vi "Asynchronous Call and Forget.vi"   [LabVIEW 2019]
doc: "This VI demonstrates an asynchronous call and forget. When this VI is run, it asynchronously calls a target VI and will not wait for the results. This VI will run to completion while the target VI continues to run.\n\nThis example uses the Start Asynchronous Call method and the Open VI Reference option 0x80.\n\nWhen running this example, notice this VI finishes execution while the target VI continues to run."
panel:
  # "Overview: Demonstrates the use of the call and forget option (0x80) with Asynchronous VI Calls.\nInstructions:\nRun the VI. Observe the behavior of the VI being called asynchronously, and notice that this VI stops running, even when the asynchronous VI is still running. See the block diagram for more information."
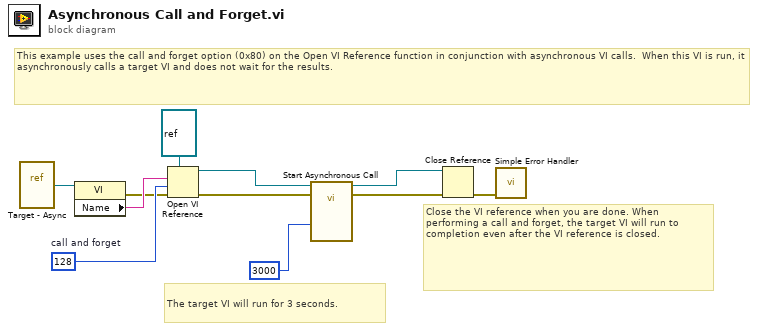
[diagram p0: block diagram]
diagram:
  w11 = 128  # call and forget
  # "This example uses the call and forget option (0x80) on the Open VI Reference function in conjunction with asynchronous VI calls.  When this VI is run, it asynchronously calls a target VI and does not wait for the results."
  # "Close the VI reference when you are done. When performing a call and forget, the target VI will run to completion even after the VI reference is closed."
  # "The target VI will run for 3 seconds."
  n1 = vi-ref "Target - Async.vi"() -> (w4:refnum<vi>)
  n2 = property class="VI"(reference=w4) -> (error out=w1:errorcluster, "Name"=w3:string)  [unwired: 1 in, 1 out]
  n3 = Open VI Reference(type specifier VI Refnum (for type only)=refnum<vi> refnum, vi path=w3, options=w11, error in (no error)=w1) -> (vi reference=w9:refnum<vi>, error out=w8:errorcluster)  [unwired: 2 in]
  n4 = call-by-ref "Start Asynchronous Call"(reference=w9, error in=w8, "Wait (ms)"=u32 3000 ("Wait (Milliseconds)")) -> (reference out=w6:refnum<vi>, error out=w7:errorcluster)  [unwired: 10 in, 1 out]
  n5 = Close Reference(reference=w6, error in (no error)=w7) -> (error out=w5:errorcluster)
  n6 = call <vilib>:"Simple Error Handler.vi"("error in (no error)"=w5) -> ()  [unwired: 4 in, 5 out]
